vi "FTW-Inbox-Core-MessageRouter.vi"(0 "ActorNotifier":refnum<user-event>, 5 "Messages from Inbox Thread":refnum<event-registration>, 7 "Routing Rules":T2[](array[typedef]) {"SendTimeout" format="%dmsec"; "BusyTimeout" format="%dmsec"}, 9 "Statistics":T1, 11 "Actor Identity":string) -> ()   [LabVIEW 2015]
uses:
  FTW-Inbox-Core-RoutingRule.ctl
  core/type/FTW-Type-JSON.ctl
  json/FTW-JSON-JoinMode.ctl
panel:
  # "Inputs"
  # "Outputs"
  # "This async worker\nhas no outputs"
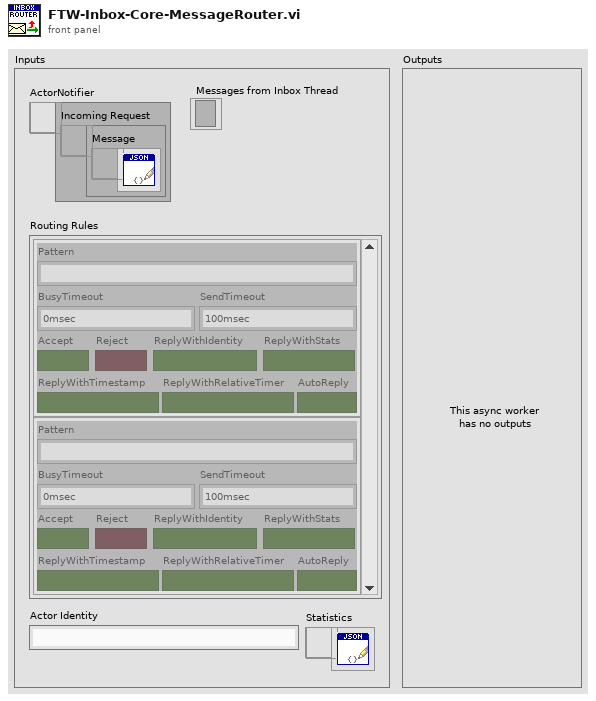
[diagram p1: front panel]
types:
  T1 = typedef "FTW-Type-JSON.ctl" = refnum<data-value>
  T2 = typedef "FTW-Inbox-Core-RoutingRule.ctl" = cluster{"Pattern":string, "BusyTimeout":i32, "SendTimeout":i32, "Accept":bool, "Reject":bool, "ReplyWithIdentity":bool, "ReplyWithStats":bool, "ReplyWithTimestamp":bool, "ReplyWithRelativeTimer":bool, "AutoReply":bool}
  T3 = cluster{"FTW-CodeGen-Type":enum16{"FTW-JSON"}, "Object":i64, "EncodingFlags":i64, "DecodingFlags":i64}
  T4 = typedef "FTW-JSON-JoinMode.ctl" = enum32{"Upsert", "Update Only", "Insert Only"}
  T5 = cluster{"Backtrace":i64, "ReplyTimeout":i32, "ReponseIncludesTimestamp":bool, "ReponseIncludesRelativeTimer":bool, "ReponseIncludesException":bool}
  T6 = typedef "FTW-JSON-Type.ctl" = enum8{"Not Found", "Object", "Array", "String", "Number", "Boolean", "null"}
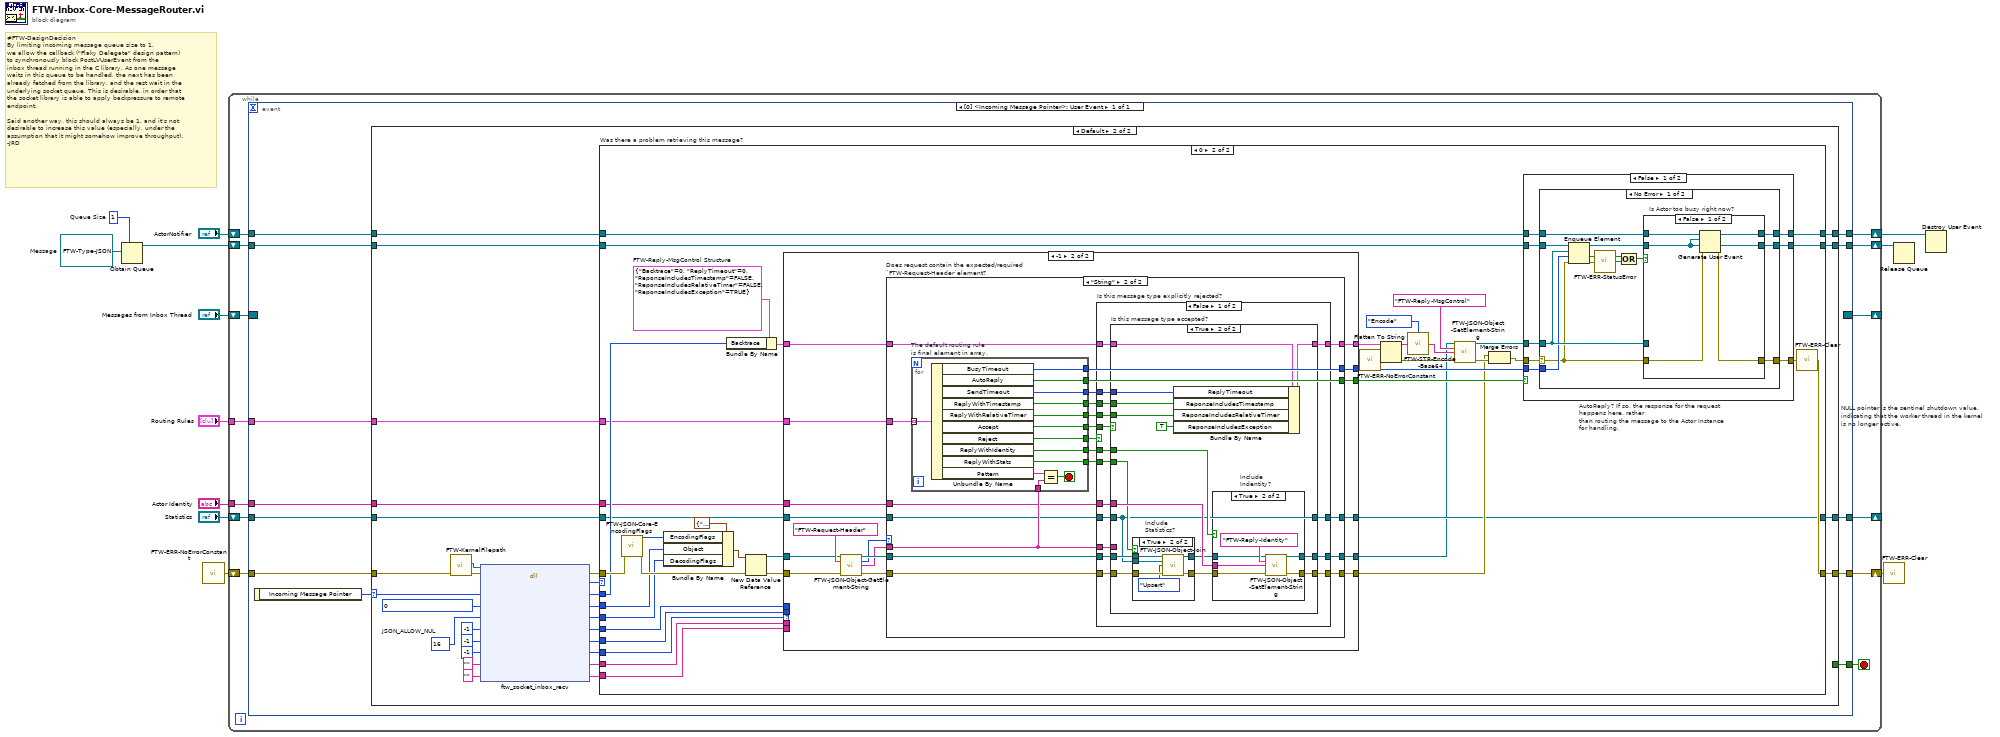
[diagram p0: block diagram]
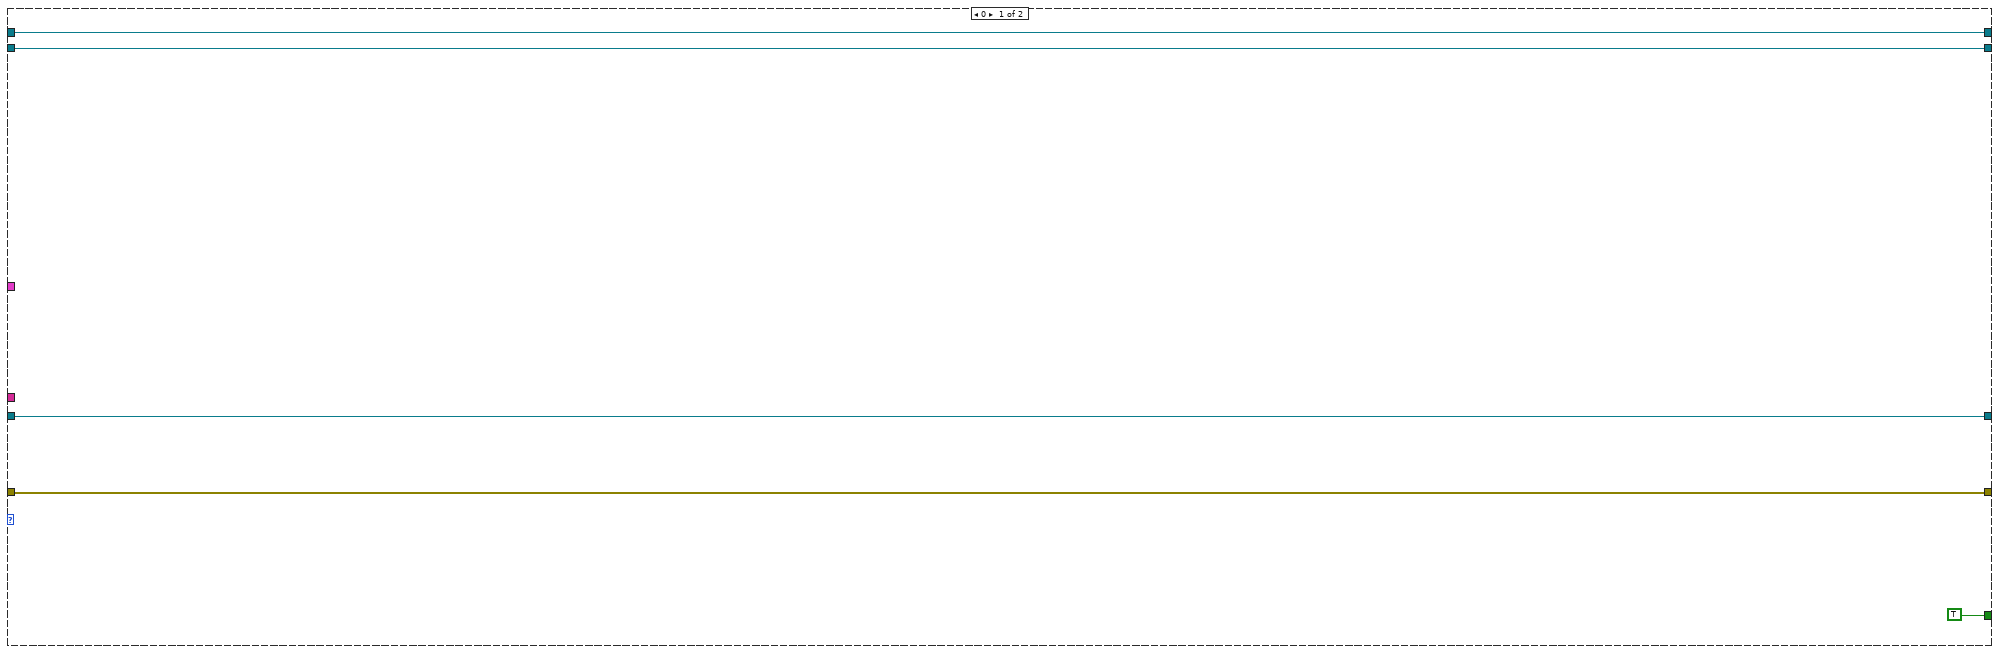
[diagram p2: hidden frame]
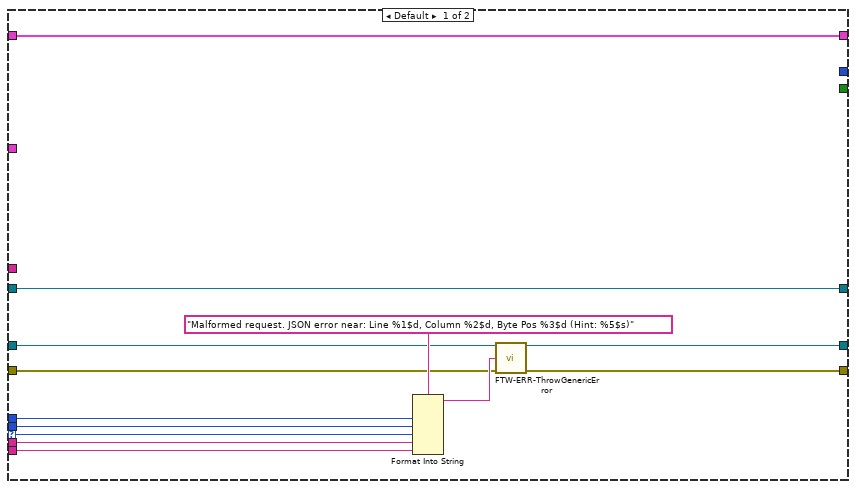
[diagram p4: hidden frame]
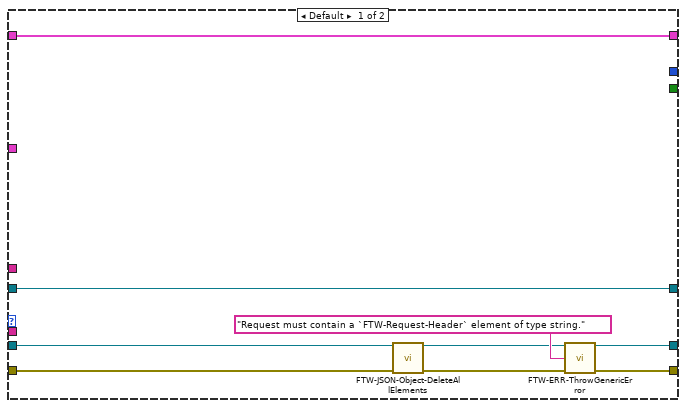
[diagram p5: hidden frame]
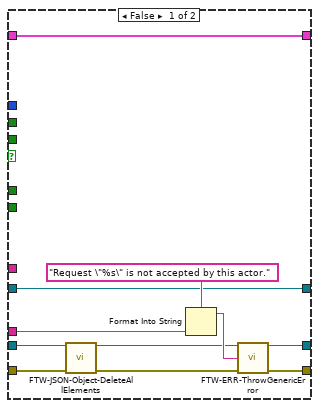
[diagram p6: hidden frame]
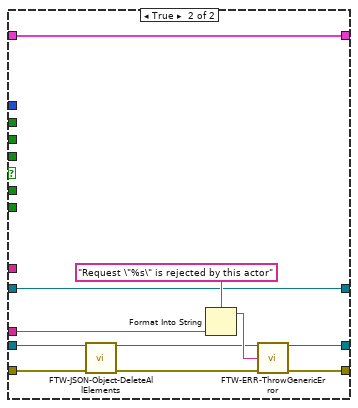
[diagram p9: hidden frame]
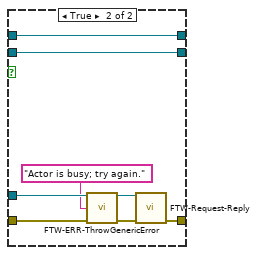
[diagram p10: hidden frame]
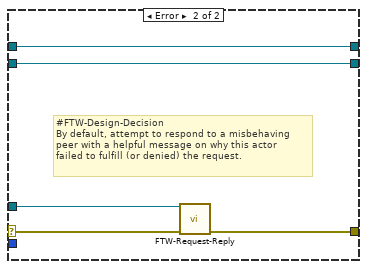
[diagram p11: hidden frame]
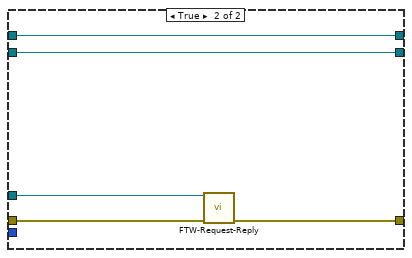
[diagram p12: hidden frame]
diagram:
  w1 = T1 refnum  # Message
  w8 = 1  # Queue Size
  # "#FTW-DesignDecision\nBy limiting incoming message queue size to 1,\nwe allow the callback (\"Flaky Delegate\" design pattern)\nto synchronously block PostLVUserEvent from the\ninbox thread running in the C library. As one message\nwaits in this queue to be handled, the next has been\nalready fetched from the library, and the rest wait in the\nunderlying socket queue. This is desirable, in order that\nthe socket library is able to apply backpressure to remote\nendpoint.\n\nSaid another way, this should always be 1, and it's not\ndesirable to increase this value (especially, under the\nassumption that it might somehow improve throughput).\n-JRD"
  n1 = Obtain Queue(max queue size (-1, unlimited)=w8, element data type=w1) -> (queue out=w7:refnum<queue>)  [unwired: 3 in, 2 out]
  n2 = call "FTW-ERR-NoErrorConstant.vi"() -> ("no error"=w4:errorcluster)
  n3 = while {
    tunnel: "Routing Rules" -> [w25]
    tunnel: "Actor Identity" -> [w24]
    shift-right: [w19] -> _
    shift-left: "Messages from Inbox Thread" -> [w20]
    shift-right: [w17] -> w6
    shift-left: w7 -> [w21]
    shift-right: [w18] -> w5
    shift-left: "ActorNotifier" -> [w22]
    shift-right: [w14] -> w3
    shift-left: w4 -> [w15]
    shift-right: [w13] -> _
    shift-left: "Statistics" -> [w23]
    stop <- w16 stop-if-true
    n4 = event shown="[0] <Incoming Message Pointer>: User Event" {
      selector: w20 -> [_]
      dyn-events: [_] -> w19
      timeout: _ -> [_]
      tunnel: [w28] -> w14
      tunnel: w25 -> [w37]
      tunnel: w24 -> [w36]
      tunnel: w23 -> [w35]
      tunnel: w22 -> [w34]
      tunnel: w21 -> [w33]
      tunnel: [w32] -> w18
      tunnel: [w31] -> w17
      tunnel: [w30] -> w16
      tunnel: w15 -> [w29]
      tunnel: [w26] -> w13
      event User Event {
        n5 = event-data() -> ("Incoming Message Pointer"=w27:i64)  [unwired: 1 in]
        n6 = case "NULL pointer is the sentinel shutdown value, indicating that the worker thread in the kernel is no longer active." shown="Default" w27 {
          selector: w27 -> [_ w47]
          tunnel: w37 -> [_ w56]
          tunnel: w36 -> [_ w55]
          tunnel: w35 -> [w38 w54]
          tunnel: w34 -> [w42 w53]
          tunnel: w33 -> [w41 w52]
          tunnel: [w42 w51] -> w32
          tunnel: [w41 w50] -> w31
          tunnel: [TRUE _] -> w30
          tunnel: w29 -> [w40 w49]
          tunnel: [w40 w48] -> w28
          tunnel: [w38 w43] -> w26
          frame 0 {
          }
          frame Default {
            w67 = i64 16  # JSON_ALLOW_NUL
            n7 = call "FTW-KernelFilepath.vi"("error in"=w49) -> ("error out"=w58:errorcluster, "Library Filepath"=w57:path)  [unwired: 8 in, 1 out]
            n8 = dll-call lib="?" fn="ftw_socket_inbox_recv"(path in=w57, error in=w58, "Message Backtrace"=w47, "JSON Object Pointer"=i64 0, "Flags"=w67, "Error Line Number"=i64 -1, "Error Column Number"=i64 -1, "Error Byte Position"=i64 -1, "Error Source"="", "Error Hint"="") -> (error out=w62:errorcluster, "JSON Object Pointer"=w44:i64, "Message Backtrace"=w59:i64, "JSON Object Pointer"=w46:i64, "Flags"=w61:i64, "Error Line Number"=w66:i64, "Error Column Number"=w65:i64, "Error Byte Position"=w60:i64, "Error Source"=w64:string, "Error Hint"=w63:string)  [unwired: 1 in, 1 out]
            n9 = case "Was there a problem retrieving this message?" shown="0" w44 {
              tunnel: w66 -> [_ w112]
              tunnel: w65 -> [_ w111]
              tunnel: w64 -> [_ w110]
              tunnel: w63 -> [_ w109]
              tunnel: w62 -> [w74 w99]
              tunnel: w61 -> [_ w98]
              tunnel: w60 -> [_ w95]
              tunnel: w59 -> [_ w94]
              tunnel: w56 -> [_ w89]
              tunnel: w55 -> [_ w88]
              tunnel: w54 -> [w73 w87]
              tunnel: w53 -> [w76 w86]
              tunnel: w52 -> [w75 w85]
              tunnel: [w76 w84] -> w51
              tunnel: [w75 w83] -> w50
              tunnel: [w74 w82] -> w48
              tunnel: w46 -> [_ w80]
              tunnel: [w73 w79] -> w43
              frame Default {
              }
              frame 0 {
                w102 = T5 {"Backtrace"=0, "ReplyTimeout"=0, "ReponseIncludesTimestamp"=FALSE, "ReponseIncludesRelativeTimer"=FALSE, "ReponseIncludesException"=TRUE}  # FTW-Reply-MsgControl Structure
                n10 = call "FTW-JSON-Core-EncodingFlags.vi"("error in"=w99) -> ("Encoding Flags"=w101:i64, "error out"=w117:errorcluster)  [unwired: 13 in]
                n11 = Bundle By Name(cluster=T3 {"FTW-CodeGen-Type"=enum."FTW-JSON", "Object"=0, "EncodingFlags"=0, "DecodingFlags"=0}, "EncodingFlags"=w101, "Object"=w80, "DecodingFlags"=w98) -> (w100:T3)
                n12 = Bundle By Name(cluster=w102, "Backtrace"=w94) -> (w108:T5)
                n13 = New Data Value Reference(data value=w100, error in=w117) -> (data value reference=w96:refnum<data-value>, error out=w97:errorcluster)
                n14 = case shown="-1" w95 {
                  selector: w95 -> [w119 _]
                  tunnel: [w121 w140] -> w90
                  tunnel: w97 -> [w127 w135]
                  tunnel: w112 -> [w126 _]
                  tunnel: w111 -> [w125 _]
                  tunnel: w110 -> [w124 _]
                  tunnel: w109 -> [w123 _]
                  tunnel: w89 -> [_ w143]
                  tunnel: [w120 w141] -> w78
                  tunnel: w108 -> [w122 w138]
                  tunnel: [w122 w139] -> w107
                  tunnel: [_ w137] -> w106
                  tunnel: w88 -> [_ w136]
                  tunnel: w96 -> [w120 w134]
                  tunnel: w87 -> [w118 w133]
                  tunnel: [_ w131] -> w93
                  tunnel: [w118 w130] -> w79
                  frame Default {
                    n15 = Format Into String(format string="Malformed request. JSON error near: Line %1$d, Column %2$d, Byte Pos %3$d (Hint: %5$s)", w126, w125, w119, w124, w123) -> (resulting string=w128:string)  [unwired: 2 in, 1 out]
                    n16 = call "FTW-ERR-ThrowGenericError.vi"("Error Message"=w128, "error in"=w127) -> ("error out"=w121:errorcluster)  [unwired: 13 in]
                  }
                  frame -1 {
                    n17 = call "FTW-JSON-Object-GetElement-String.vi"("JSON"=w134, "Key"="FTW-Request-Header", "error in"=w135) -> ("JSON out"=w144:T1, "JSON Element Type"=w132:T6, "Value"=w142:string, "error out"=w145:errorcluster)  [unwired: 9 in]
                    n18 = case "Does request contain the expected/required `FTW-Request-Header`element?" shown="\"String\"" w132 {
                      tunnel: w145 -> [w150 w174]
                      tunnel: w144 -> [w152 w173]
                      tunnel: [w151 w167] -> w141
                      tunnel: [w153 w172] -> w140
                      tunnel: w143 -> [_ w171]
                      tunnel: w142 -> [_ w168]
                      tunnel: [w148 w165] -> w139
                      tunnel: w138 -> [w148 w166]
                      tunnel: [_ w161] -> w137
                      tunnel: w136 -> [_ w160]
                      tunnel: w133 -> [w147 w159]
                      tunnel: [_ w156] -> w131
                      tunnel: [w147 w155] -> w130
                      frame Default {
                        n19 = call "FTW-JSON-Object-DeleteAllElements.vi"("JSON"=w152, "error in"=w150) -> ("JSON out"=w151:T1, "error out"=w149:errorcluster)  [unwired: 12 in]
                        n20 = call "FTW-ERR-ThrowGenericError.vi"("Error Message"="Request must contain a `FTW-Request-Header` element of type string.", "error in"=w149) -> ("error out"=w153:errorcluster)  [unwired: 13 in]
                      }
                      frame "String" {
                        n21 = for "The default routing rule is final element in array." {
                          tunnel: w171 -> [w255] mode=indexing
                          tunnel: w168 -> [w253]
                          tunnel: [w247] -> w170
                          tunnel: [w248] -> w169
                          tunnel: [w251] -> w164
                          tunnel: [w250] -> w163
                          tunnel: [w249] -> w162
                          tunnel: [w244] -> w161
                          tunnel: [w246] -> w158
                          tunnel: [w245] -> w157
                          tunnel: [w243] -> w156
                          stop <- w252 stop-if-true
                          n22 = Unbundle By Name(w255) -> ("BusyTimeout"=w244:i32, "AutoReply"=w243:bool, "SendTimeout"=w249:i32, "ReplyWithTimestamp"=w250:bool, "ReplyWithRelativeTimer"=w251:bool, "Accept"=w248:bool, "Reject"=w247:bool, "ReplyWithIdentity"=w246:bool, "ReplyWithStats"=w245:bool, "Pattern"=w254:string)
                          n23 = Equal?(x=w254, y=w253) -> (x = y?=w252:bool)
                        }
                        n24 = case "Is this message type explicitly rejected?" shown="False" w170 {
                          tunnel: w174 -> [w190 w237]
                          tunnel: w173 -> [w189 w238]
                          tunnel: [w188 w242] -> w172
                          tunnel: w169 -> [w187 _]
                          tunnel: w168 -> [w185 w239]
                          tunnel: [w186 w235] -> w167
                          tunnel: w166 -> [w184 w234]
                          tunnel: [w183 w234] -> w165
                          tunnel: w164 -> [w182 _]
                          tunnel: w163 -> [w181 _]
                          tunnel: w162 -> [w180 _]
                          tunnel: w160 -> [w179 _]
                          tunnel: w159 -> [w178 w233]
                          tunnel: w158 -> [w177 _]
                          tunnel: w157 -> [w176 _]
                          tunnel: [w175 w233] -> w155
                          frame False {
                            n25 = case "Is this message type accepted?" shown="True" w187 {
                              tunnel: w190 -> [w197 w202]
                              tunnel: w189 -> [w199 w206]
                              tunnel: [w194 w209] -> w188
                              tunnel: [w198 w210] -> w186
                              tunnel: w185 -> [w193 _]
                              tunnel: w184 -> [w192 w216]
                              tunnel: [w192 w215] -> w183
                              tunnel: w182 -> [_ w214]
                              tunnel: w181 -> [_ w211]
                              tunnel: w180 -> [_ w213]
                              tunnel: w179 -> [_ w208]
                              tunnel: w178 -> [w191 w201]
                              tunnel: w177 -> [_ w207]
                              tunnel: w176 -> [_ w205]
                              tunnel: [w191 w201] -> w175
                              frame False {
                                n26 = call "FTW-JSON-Object-DeleteAllElements.vi"("JSON"=w199, "error in"=w197) -> ("JSON out"=w198:T1, "error out"=w195:errorcluster)  [unwired: 12 in]
                                n27 = Format Into String(format string="Request \"%s\" is not accepted by this actor." ("Error Message"), w193) -> (resulting string=w200:string)  [unwired: 2 in, 1 out]
                                n28 = call "FTW-ERR-ThrowGenericError.vi"("Error Message"=w200, "error in"=w195) -> ("error out"=w194:errorcluster)  [unwired: 13 in]
                              }
                              frame True {
                                n29 = case "Include\nStatistics?" shown="True" w205 {
                                tunnel: w206 -> [w218 w224]
                                tunnel: [w218 w223] -> w204
                                tunnel: [w217 w220] -> w203
                                tunnel: w202 -> [w217 w221]
                                tunnel: w201 -> [_ w222]
                                frame False {
                                }
                                frame True {
                                n30 = call "FTW-JSON-Object-Join.vi"("JSON"=w224, "JSON to Join"=w222, "Join Mode"=FTW-JSON-JoinMode."Upsert", "error in"=w221) -> ("JSON out"=w223:T1, "error out"=w220:errorcluster)  [unwired: 10 in]
                                }
                                }
                                n31 = Bundle By Name(cluster=w216, "ReplyTimeout"=w213, "ReponseIncludesTimestamp"=w211, "ReponseIncludesRelativeTimer"=w214, "ReponseIncludesException"=TRUE) -> (w215:T5)
                                n32 = case "Include\nIndentity?" shown="True" w207 {
                                tunnel: w204 -> [w226 w231]
                                tunnel: [w226 w230] -> w210
                                tunnel: [w225 w229] -> w209
                                tunnel: w203 -> [w225 w228]
                                tunnel: w208 -> [_ w227]
                                frame False {
                                }
                                frame True {
                                n33 = call "FTW-JSON-Object-SetElement-String.vi"("JSON"=w231, "Key"="FTW-Reply-Identity", "Value"=w227, "error in"=w228) -> ("JSON out"=w230:T1, "error out"=w229:errorcluster)  [unwired: 10 in]
                                }
                                }
                              }
                            }
                          }
                          frame True {
                            n34 = call "FTW-JSON-Object-DeleteAllElements.vi"("JSON"=w238, "error in"=w237) -> ("JSON out"=w235:T1, "error out"=w236:errorcluster)  [unwired: 12 in]
                            n35 = Format Into String(format string="Request \"%s\" is rejected by this actor" ("Error Message"), w239) -> (resulting string=w241:string)  [unwired: 2 in, 1 out]
                            n36 = call "FTW-ERR-ThrowGenericError.vi"("Error Message"=w241, "error in"=w236) -> ("error out"=w242:errorcluster)  [unwired: 13 in]
                          }
                        }
                      }
                    }
                  }
                }
                n37 = call "FTW-ERR-NoErrorConstant.vi"() -> ("no error"=w104:errorcluster)
                n38 = Flatten To String(anything=w107, error in (no error)=w104) -> (data string=w115:string, error out=w105:errorcluster)  [unwired: 2 in, 1 out]
                n39 = call "FTW-STR-Encode-Base64.vi"("Input"=w115, "Direction"=enum16{"Encode", "Decode"}."Encode") -> ("Output"=w113:string)
                n40 = call "FTW-JSON-Object-SetElement-String.vi"("JSON"=w78, "Key"="FTW-Reply-MsgControl", "Value"=w113, "error in"=w105) -> ("JSON out"=w92:T1, "error out"=w91:errorcluster)  [unwired: 10 in]
                n41 = Merge Errors(w90, w91) -> (w103:errorcluster)
                n42 = case "AutoReply? If so, the response for the request happens here, rather\nthan routing the message to the Actor Instance for handling." shown="False" w93 {
                  tunnel: [w263 w296] -> w81
                  tunnel: w106 -> [w262 _]
                  tunnel: w85 -> [w261 w295]
                  tunnel: w86 -> [w260 w294]
                  tunnel: w103 -> [w259 w297]
                  tunnel: w92 -> [w258 w298]
                  tunnel: [w257 w294] -> w84
                  tunnel: [w256 w295] -> w83
                  frame False {
                    n43 = case shown="No Error" w259 {
                      selector: w259 -> [w266 w292]
                      tunnel: w258 -> [w276 w293]
                      tunnel: w262 -> [w275 _]
                      tunnel: [w274 w291] -> w263
                      tunnel: w261 -> [w269 w289]
                      tunnel: w260 -> [w268 w290]
                      tunnel: [w265 w290] -> w257
                      tunnel: [w264 w289] -> w256
                      frame No Error {
                        n44 = Enqueue Element(queue=w269, element=w276, timeout in ms (-1)=w275, error in (no error)=w266) -> (queue out=w273:refnum<queue>, timed out?=w272:bool, error out=w270:errorcluster)
                        n45 = call "FTW-ERR-StatusError.vi"("error to check"=w270) -> ("Error?"=w267:bool)
                        n46 = Compound Arithmetic op=OR(w272, w267) -> (w271:bool)
                        n47 = case "Is Actor too busy right now?" shown="False" w271 {
                          tunnel: [w281 w288] -> w274
                          tunnel: w268 -> [w280 w282]
                          tunnel: w266 -> [w279 w286]
                          tunnel: w273 -> [w277 w283]
                          tunnel: w276 -> [_ w287]
                          tunnel: [w278 w282] -> w265
                          tunnel: [w277 w283] -> w264
                          frame False {
                            n48 = Generate User Event(user event=w280, event data cluster=w277, error in=w279) -> (user event out=w278:refnum<user-event>, error out=w281:errorcluster)  [unwired: 1 in]
                          }
                          frame True {
                            n49 = call "FTW-ERR-ThrowGenericError.vi"("Error Message"="Actor is busy; try again.", "error in"=w286) -> ("error out"=w285:errorcluster)  [unwired: 13 in]
                            n50 = call "FTW-Request-Reply.vi"("Request"=w287, "error in"=w285) -> ("error out"=w288:errorcluster)  [unwired: 13 in]
                          }
                        }
                      }
                      frame Error {
                        # "#FTW-Design-Decision\nBy default, attempt to respond to a misbehaving\npeer with a helpful message on why this actor\nfailed to fulfill (or denied) the request."
                        n51 = call "FTW-Request-Reply.vi"("Request"=w293, "error in"=w292) -> ("error out"=w291:errorcluster)  [unwired: 13 in]
                      }
                    }
                  }
                  frame True {
                    n52 = call "FTW-Request-Reply.vi"("Request"=w298, "error in"=w297) -> ("error out"=w296:errorcluster)  [unwired: 13 in]
                  }
                }
                n53 = call "FTW-ERR-Clear.vi"("error to snuff"=w81) -> ("no error"=w82:errorcluster)
              }
            }
          }
        }
      }
    }
  }
  n54 = call "FTW-ERR-Clear.vi"("error to snuff"=w3) -> ()  [unwired: 1 out]
  n55 = Release Queue(queue=w6) -> ()  [unwired: 2 in, 3 out]
  n56 = Destroy User Event(user event=w5) -> ()  [unwired: 1 in, 1 out]
